vi "main_value11.vi"(0 "values":i16[](array[numeric]), 1 "q":i32[](array[numeric])) -> (2 "main":dbl, 4 "hist":cluster{sgl[], "q":i32[]})   [LabVIEW 2010]
panel:
  # "Вычисление главного значения по трем наиболее часто встречающимся значениям."
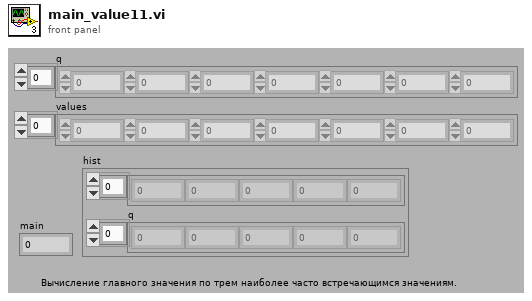
[diagram p1: front panel]
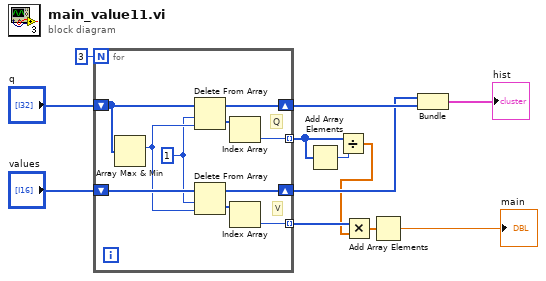
[diagram p0: block diagram]
diagram:
  n1 = for {
    N: 3 -> [_]
    shift-right: [w21] -> w8
    shift-left: "q" -> [w22]
    tunnel: [w14] -> w12 mode=indexing
    tunnel: [w13] -> w4 mode=indexing
    shift-right: [w18] -> w7
    shift-left: "values" -> [w19]
    w15 = 1 ("length")
    # "V"
    # "Q"
    n2 = Array Max & Min(array=w22) -> (max index (indices)=w17:i32)  [unwired: 3 out]
    n3 = Delete From Array(array=w22, length=w15, index=w17) -> (deleted portion=w20:i32[], array with subset deleted=w21:i32[])
    n4 = Delete From Array(array=w19, length=w15, index=w17) -> (deleted portion=w16:i16[], array with subset deleted=w18:i16[])
    n5 = Index Array(array=w20) -> (element=w13:i32)  [unwired: 1 in]
    n6 = Index Array(array=w16) -> (element=w14:i16)  [unwired: 1 in]
  }
  n7 = Add Array Elements(numeric array=w4) -> (sum=w10:i32)
  n8 = Divide(x=w4, y=w10) -> (x/y=w2:dbl[])
  n9 = Multiply(x=w12, y=w2) -> (x*y=w3:dbl[])
  n10 = Add Array Elements(numeric array=w3) -> (sum=→"main":dbl)
  n11 = Bundle("values"=w7, "q"=w8) -> (→"hist":cluster{"values":i16[], "q":i32[]})  [unwired: 1 in]
